vi "excecute.vi"(8 "error in (no error)":errorcluster, 11 "command in":refnum<class "command_click.lvclass">) -> (0 "error out":errorcluster, 3 "command out":refnum<class "command_click.lvclass">)   [LabVIEW 2015]
uses:
  canon_m3/command_click.lvclass
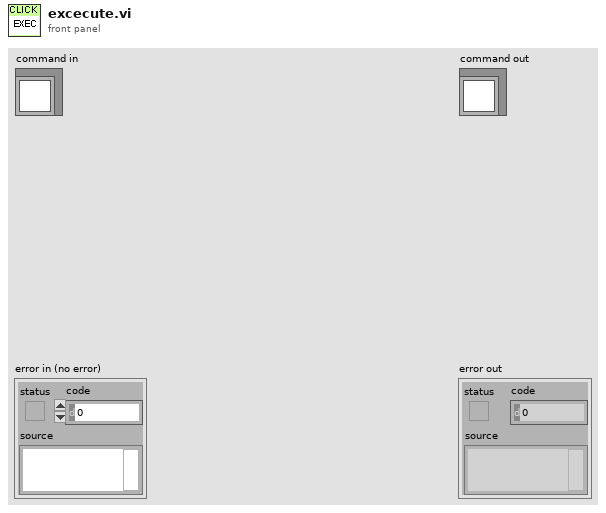
[diagram p1: front panel]
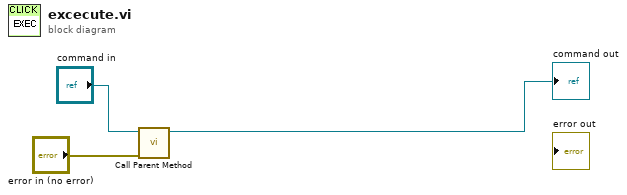
[diagram p0: block diagram]
diagram:
  n1 = call-parent "Call Parent Method"("error in (no error)"="error in (no error)", "command in"="command in") -> ("command out"=→"command out":refnum<class "command_click.lvclass">)  [unwired: 8 in, 1 out]
